vi "PH_PSDBWriter.write Datasets.vi"(1 "PSDB Credentials":T1={"PW"="N/A", "ID"="N/A", "DS"="N/A"}, 2 "Shot #":i32, 3 "Datasets":cluster{"ID":i32, "Data":T2}[](array[cluster]), 5 "error in (no error)":errorcluster) -> (19 "error out":errorcluster)   [LabVIEW 2014, in "PH_PSDBWriter.lvlib"]
uses:
  PH_PSDBWriter.lvlib
  PH_PSDBWriter.PSDB Dataset.ctl
  PH_PSDBWriter.2D dataset.ctl
  CSlibraries-extern/psdb_lv/PSDB_AxisDescription.ctl
  PH_PSDBWriter.Boolean dataset.ctl
  PH_PSDBWriter.Image dataset.ctl
  <vilib>/vision/Image Controls.llb/IMAQ Image.ctl
  PH_PSDBWriter.Numeric dataset.ctl
  PH_PSDBWriter.String dataset.ctl
  PH_Common/Connection/PH_Connection.PSDB Credentials.ctl
  CSlibraries-extern/psdb_lv/PSDB_SetInstanceValue(2dData).vi
  CSlibraries-extern/psdb_lv/PSDB_SetInstanceValue(Boolean).vi
  CSlibraries-extern/psdb_lv/PSDB_SetInstanceValue(Image).vi
  CSlibraries-extern/psdb_lv/PSDB_SetInstanceValue(Numeric).vi
  CSlibraries-extern/psdb_lv/PSDB_SetInstanceValue(String).vi
  CSlibraries-extern/psdb_lv/PSDB.lvlib
  PH_Common/PH_Common.lvlib
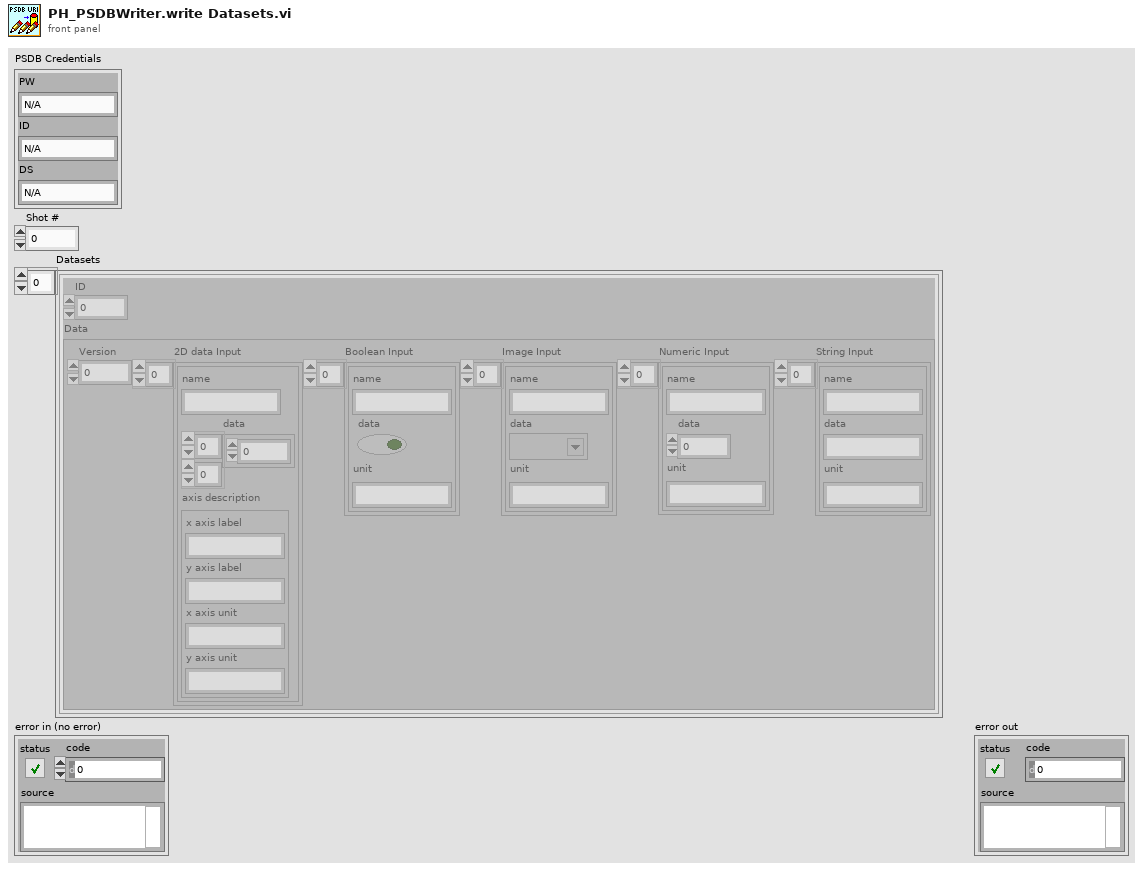
[diagram p1: front panel]
types:
  T1 = typedef "PH_Common.lvlib/PH_Connection.PSDB Credentials.ctl" = cluster{"PW":string, "ID":string, "DS":string}
  T2 = typedef "PH_PSDBWriter.lvlib/PH_PSDBWriter.PSDB Dataset.ctl" = cluster{"Version":i32, "2D data Input":T3[], "Boolean Input":T5[], "Image Input":T6[], "Numeric Input":T8[], "String Input":T9[]}
  T3 = typedef "PH_PSDBWriter.lvlib/PH_PSDBWriter.2D dataset.ctl" = cluster{"name":string, "data":dbl[][], "axis description":T4}
  T4 = typedef "PSDB.lvlib/PSDB_AxisDescription.ctl" = cluster{"x axis label":string, "y axis label":string, "x axis unit":string, "y axis unit":string}
  T5 = typedef "PH_PSDBWriter.lvlib/PH_PSDBWriter.Boolean dataset.ctl" = cluster{"name":string, "data":bool, "unit":string}
  T6 = typedef "PH_PSDBWriter.lvlib/PH_PSDBWriter.Image dataset.ctl" = cluster{"name":string, "data":T7, "unit":string}
  T7 = typedef "IMAQ Image.ctl" = refnum<image>
  T8 = typedef "PH_PSDBWriter.lvlib/PH_PSDBWriter.Numeric dataset.ctl" = cluster{"name":string, "data":dbl, "unit":string}
  T9 = typedef "PH_PSDBWriter.lvlib/PH_PSDBWriter.String dataset.ctl" = cluster{"name":string, "data":string, "unit":string}
  T10 = typedef "NI_Database_API.lvlib/Conn ObjectReference.ctl" = refnum<k1>
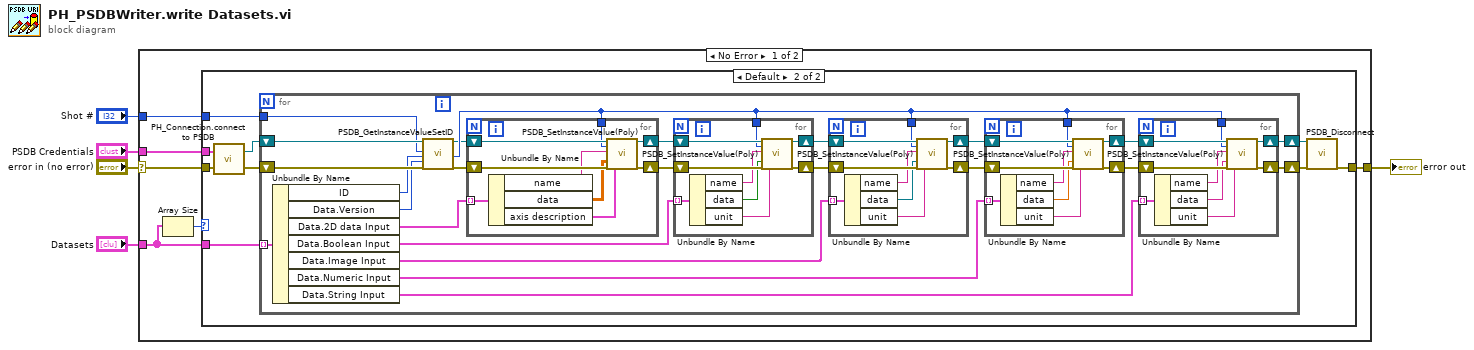
[diagram p0: block diagram]
diagram:
  n1 = case shown="No Error" "error in (no error)" {
    selector: "error in (no error)" -> [w9 w91]
    tunnel: [w11 w91] -> w5
    tunnel: "Shot #" -> [w10 _]
    tunnel: "Datasets" -> [w7 _]
    tunnel: "PSDB Credentials" -> [w6 _]
    frame No Error {
      n2 = Array Size(array=w7) -> (size(s)=w8:i32)
      n3 = case shown="Default" w8 {
        tunnel: [w12 w21] -> w11
        tunnel: w10 -> [_ w16]
        tunnel: w7 -> [_ w15]
        tunnel: w9 -> [w12 w14]
        tunnel: w6 -> [_ w13]
        frame 0 {
        }
        frame Default {
          n4 = call "PH_Connection.connect to PSDB.vi"("error in"=w14, "PSDB Credentials"=w13) -> ("error out"=w17:errorcluster, "connection reference"=w18:T10)
          n5 = for {
            tunnel: w16 -> [w30]
            tunnel: w15 -> [w29] mode=indexing
            shift-right: [w43] -> w20
            shift-left: w18 -> [w32]
            shift-right: [w42] -> w19
            shift-left: w17 -> [w31]
            n6 = Unbundle By Name(w29) -> ("ID"=w22:i32, "Data.Version"=w23:i32, "Data.2D data Input"=w24:T3[], "Data.Boolean Input"=w25:T5[], "Data.Image Input"=w26:T6[], "Data.Numeric Input"=w27:T8[], "Data.String Input"=w28:T9[])
            n7 = call "PSDB_GetInstanceValueSetID.vi"("connection reference"=w32, "shot_id"=w30, "instance_id"=w22, "version (0)"=w23, "error in (no error)"=w31) -> ("connection reference out"=w34:T10, "instancevalueset_id"=w44:i32, "error out"=w33:errorcluster)  [unwired: 12 in]
            n8 = for {
              tunnel: w44 -> [w86]
              shift-right: [w87] -> w45
              shift-left: w34 -> [w88]
              shift-right: [w89] -> w35
              shift-left: w33 -> [w90]
              tunnel: w24 -> [w85] mode=indexing
              n9 = Unbundle By Name(w85) -> ("name"=w84:string, "data"=w83:dbl[][], "axis description"=w82:T4)
              n10 = call-poly "PSDB_SetInstanceValue(Poly).vi"("connection reference"=w88, "instancevalueset_id"=w86, "name"=w84, "data"=w83, "error in (no error)"=w90, "axis description"=w82) -> ("connection reference out"=w87:T10, "error out"=w89:errorcluster)  [unwired: 12 in]
            }
            n11 = for {
              tunnel: w44 -> [w77]
              shift-right: [w78] -> w37
              shift-left: w45 -> [w79]
              shift-right: [w80] -> w36
              shift-left: w35 -> [w81]
              tunnel: w25 -> [w76] mode=indexing
              n12 = Unbundle By Name(w76) -> ("name"=w75:string, "data"=w74:bool, "unit"=w73:string)
              n13 = call-poly "PSDB_SetInstanceValue(Poly).vi"("connection reference"=w79, "instancevalueset_id"=w77, "name"=w75, "data"=w74, "error in (no error)"=w81, "unit"=w73) -> ("connection reference out"=w78:T10, "error out"=w80:errorcluster)  [unwired: 12 in]
            }
            n14 = for {
              tunnel: w44 -> [w68]
              shift-right: [w69] -> w38
              shift-left: w37 -> [w70]
              shift-right: [w71] -> w39
              shift-left: w36 -> [w72]
              tunnel: w26 -> [w67] mode=indexing
              n15 = Unbundle By Name(w67) -> ("name"=w66:string, "data"=w65:T7, "unit"=w64:string)
              n16 = call-poly "PSDB_SetInstanceValue(Poly).vi"("connection reference"=w70, "instancevalueset_id"=w68, "name"=w66, "data"=w65, "error in (no error)"=w72, "unit"=w64) -> ("connection reference out"=w69:T10, "error out"=w71:errorcluster)  [unwired: 12 in]
            }
            n17 = for {
              tunnel: w44 -> [w59]
              shift-right: [w60] -> w41
              shift-left: w38 -> [w61]
              shift-right: [w62] -> w40
              shift-left: w39 -> [w63]
              tunnel: w27 -> [w58] mode=indexing
              n18 = Unbundle By Name(w58) -> ("name"=w57:string, "data"=w56:dbl, "unit"=w55:string)
              n19 = call-poly "PSDB_SetInstanceValue(Poly).vi"("connection reference"=w61, "instancevalueset_id"=w59, "name"=w57, "data"=w56, "error in (no error)"=w63, "unit"=w55) -> ("connection reference out"=w60:T10, "error out"=w62:errorcluster)  [unwired: 12 in]
            }
            n20 = for {
              tunnel: w44 -> [w50]
              shift-right: [w51] -> w43
              shift-left: w41 -> [w52]
              shift-right: [w53] -> w42
              shift-left: w40 -> [w54]
              tunnel: w28 -> [w49] mode=indexing
              n21 = Unbundle By Name(w49) -> ("name"=w48:string, "data"=w47:string, "unit"=w46:string)
              n22 = call-poly "PSDB_SetInstanceValue(Poly).vi"("connection reference"=w52, "instancevalueset_id"=w50, "name"=w48, "data"=w47, "error in (no error)"=w54, "unit"=w46) -> ("connection reference out"=w51:T10, "error out"=w53:errorcluster)  [unwired: 12 in]
            }
          }
          n23 = call "PSDB_Disconnect.vi"("connection reference"=w20, "error in (no error)"=w19) -> ("error out"=w21:errorcluster)  [unwired: 17 in]
        }
      }
    }
    frame Error {
    }
  }
  "error out" <- w5
